vi "Proyecto_Instrumentacion_sensores.vi"() -> ()   [LabVIEW 2020]
uses:
  <vilib>/Instr/_visa.llb/VISA Configure Serial Port (Instr).vi
panel:
  out "Presion":dbl format="%#_10g"
  out "Gas_Ambiente":dbl
  out "TemperaturaAmbiente_LM35":dbl format="%#_10g"
  out "HumedadAmbiente_AHT20":dbl format="%#_10g"
  out "% HumedadTierra_HL69":dbl format="%#_10g"
  out "HumedadTierra_HL69":dbl format="%#_10g"
  out "Sensor_Del_Gas":bool
  out "Fuera del Rango.":bool
  in  "Puerto COM a elegir":refnum<visa-resource-name>
  out "Datos mostrados":refnum<visa-resource-name>
  in  "Min_P1":dbl
  in  "Max_P1":dbl
  in  "Min_P2":dbl
  in  "Max_P2":dbl
  in  "Cambio\nde Perfil":bool
  in  "Max_Gas":dbl
  in  "?":bool
  # "Pefiles de plantas"
  # "Malamadre"
  # "Savila"
  # "UNIDAD PROFESIONAL INTERDISCIPLINARIA \nDE INGENIERIA CAMPUS ZACATECAS"
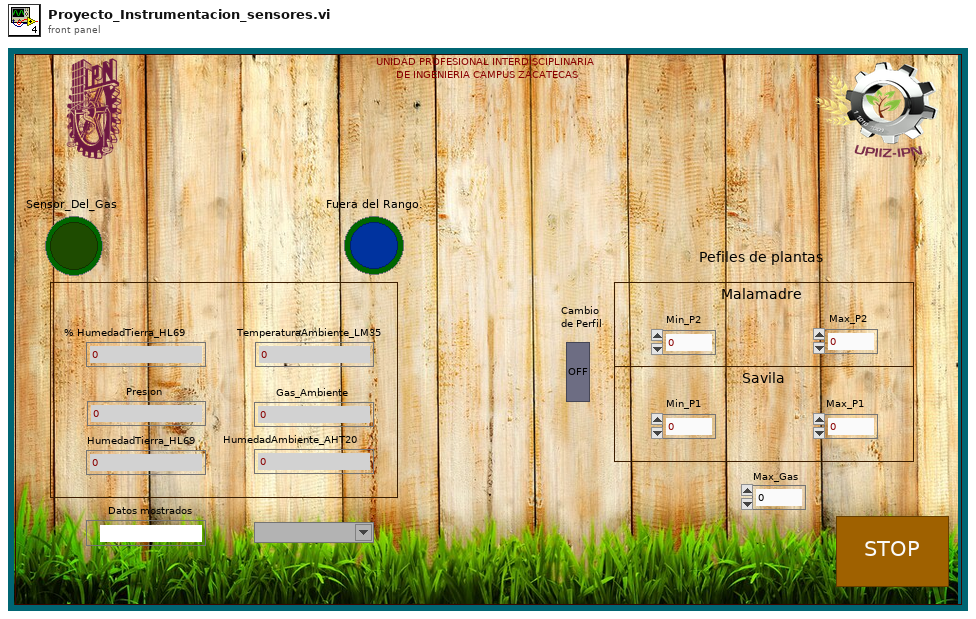
[diagram p1: front panel]
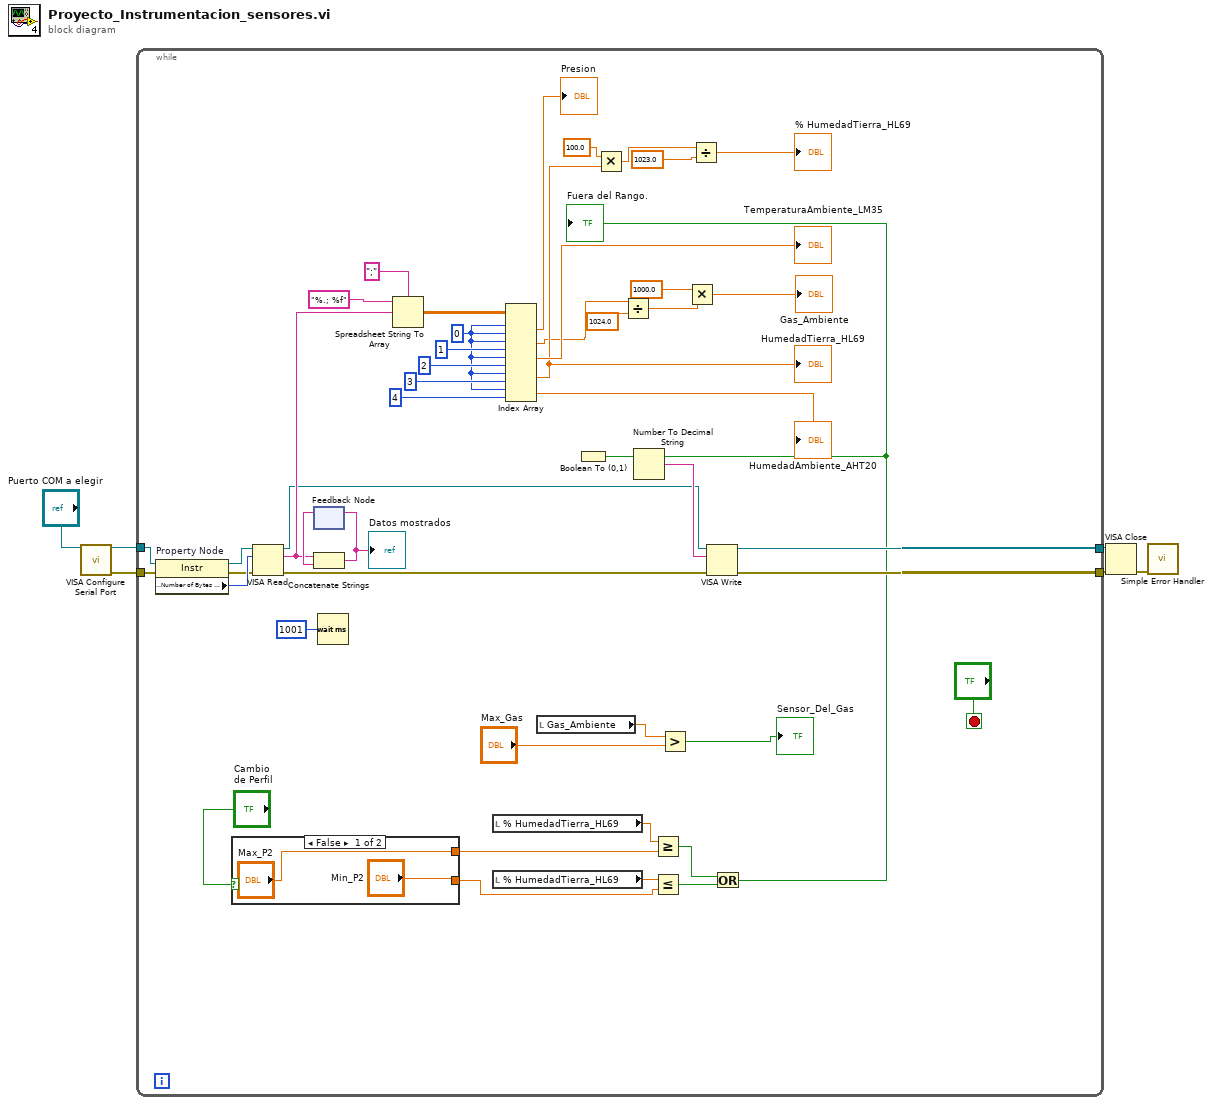
[diagram p0: block diagram]
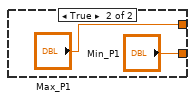
[diagram p2: hidden frame]
diagram:
  n1 = call-poly "VISA Configure Serial Port"("VISA resource name"="Puerto COM a elegir") -> ("VISA resource name out"=w2:refnum<visa-resource-name>, "error out"=w3:errorcluster)  [unwired: 13 in]
  n2 = while {
    tunnel: w2 -> [w54]
    tunnel: w3 -> [w53]
    tunnel: [w27] -> w6
    tunnel: [w29] -> w5
    stop <- "?" stop-if-true
    w23 = 0 ("index (row)")
    n3 = property on="Property Node" class="Instr"(reference=w54, error in=w53) -> (reference out=w51:refnum<visa-resource-name>, error out=w50:errorcluster, "Serial Settings:Number of Bytes at Serial Port"=w52:u32)
    n4 = case shown="False" "Cambio\nde Perfil" {
      tunnel: ["Max_P2" "Max_P1"] -> w11
      tunnel: ["Min_P2" "Min_P1"] -> w10
      frame False {
      }
      frame True {
      }
    }
    n5 = VISA Read(VISA resource name=w51, byte count=w52, error in (no error)=w50) -> (VISA resource name out=w30:refnum<visa-resource-name>, read buffer=w41:string, error out=w28:errorcluster)  [unwired: 1 out]
    n6 = feedback #1() -> (w42:string)  [unwired: 1 in]
    n7 = Concatenate Strings(w41, w42) -> (w40:string)
    "Datos mostrados" <- w40
    n8 = feedback-in #1(w40) -> ()
    n9 = Wait (ms)(milliseconds to wait=u32 1001) -> ()  [unwired: 1 out]
    n10 = Spreadsheet String To Array(delimiter (Tab)=";", format string="%.; %f", spreadsheet string=w41) -> (array=w43:dbl[][])  [unwired: 1 in]
    n11 = local read "% HumedadTierra_HL69"() -> (w33:dbl)
    n12 = local read "% HumedadTierra_HL69"() -> (w32:dbl)
    n13 = Index Array(array=w43, index (row) #1=w23, index (col) #1=w23, index (row) #2=w23, index (col) #2=1 ("index (col)"), index (row) #3=w23, index (col) #3=2 ("index (col)"), index (row) #4=w23, index (col) #4=3 ("disabled index (col)"), index (row) #5=w23, index (col) #5=4 ("disabled index (col)")) -> (element #1=→"Presion":dbl, element #2=w18:dbl, element #3=→"TemperaturaAmbiente_LM35":dbl, element #4=w20:dbl, element #5=→"HumedadAmbiente_AHT20":dbl)
    "HumedadTierra_HL69" <- w20
    n14 = local read "Gas_Ambiente"() -> (w9:dbl)
    n15 = Multiply(x=100.0, y=w20) -> (x*y=w38:dbl)
    n16 = Divide(x=w18, y=1024.0) -> (x/y=w16:dbl)
    n17 = Greater Or Equal?(x=w33, y=w11) -> (x >= y?=w35:bool)
    n18 = Less Or Equal?(x=w32, y=w10) -> (x <= y?=w34:bool)
    n19 = Greater?(x=w9, y="Max_Gas") -> (0:→"Sensor_Del_Gas":bool)
    n20 = Multiply(x=1000.0, y=w16) -> (x*y=→"Gas_Ambiente":dbl)
    n21 = Divide(x=w38, y=1023.0) -> (x/y=→"% HumedadTierra_HL69":dbl)
    n22 = Or(x=w35, y=w34) -> (x .or. y?=w26:bool)
    "Fuera del Rango." <- w26
    n23 = Boolean To (0,1)(Boolean=w26) -> (0, 1=w25:i16)
    n24 = Number To Decimal String(number=w25) -> (decimal integer string=w31:string)  [unwired: 1 in]
    n25 = VISA Write(VISA resource name=w30, write buffer=w31, error in (no error)=w28) -> (VISA resource name out=w29:refnum<visa-resource-name>, error out=w27:errorcluster)  [unwired: 1 out]
  }
  n26 = VISA Close(VISA resource name=w5, error in (no error)=w6) -> (error out=w4:errorcluster)
  n27 = call <vilib>:"Simple Error Handler.vi"("error in (no error)"=w4) -> ()  [unwired: 4 in, 5 out]
